vi "DrawTextOnMinMaxPlot.vi"(1 "[user-specified font]":T1={"Font Name:"="Current Font", "Size"=36, "Strikeout?"=FALSE, "Italic?"=FALSE, "Underline?"=FALSE, "Outline?"=TRUE, "Shadow?"=TRUE, "Bold?"=TRUE}, 2 "desired font(Application)":T2(ring), 3 "Text To Draw":string, 4 "Min Max Plot In":picture) -> (0 "Min Max Plot Out":picture)   [LabVIEW 2011]
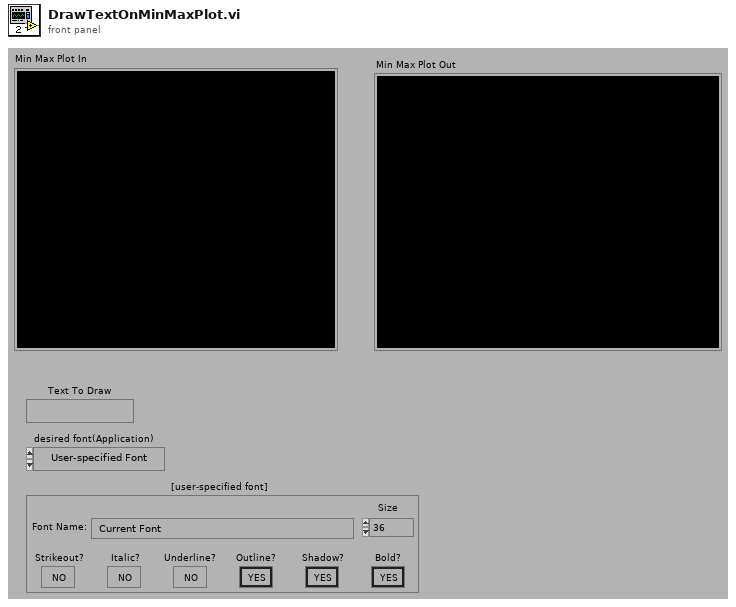
[diagram p1: front panel]
types:
  T1 = cluster{"Font Name:":string, "Size":i16, "Strikeout?":bool, "Italic?":bool, "Underline?":bool, "Outline?":bool, "Shadow?":bool, "Bold?":bool}
  T2 = enum16{"User-specified Font", "Application Font", "System Font", "Dialog Font"}
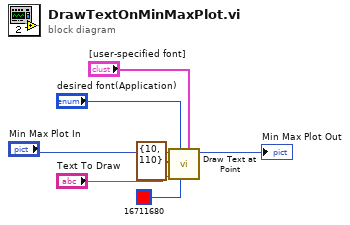
[diagram p0: block diagram]
diagram:
  n1 = call <vilib>:"Draw Text at Point.vi"("[user-specified font]"="[user-specified font]", "text color(black)"=u32 16711680, "desired font(Application)"="desired font(Application)", "text"="Text To Draw", "origin"=cluster{"x":i16, "y":i16} {"x"=10, "y"=110}, "picture"="Min Max Plot In") -> ("new picture"=→"Min Max Plot Out":picture)  [unwired: 3 in, 2 out]
